vi "Exercise 4.4.vi"() -> ()   [LabVIEW 2020]
uses:
  <vilib>/Analysis/NI_AALBase.lvlib
  <vilib>/Analysis/3filter.llb/Butterworth Filter (DBL).vi
  <vilib>/Analysis/3filter.llb/Filter Passband Type.ctl
panel:
  in  "high cutoff freq: fh":dbl=39.0 format="%0.2f"
  in  "low cutoff freq:":dbl=39.105000000000004 format="%0.4f"
  in  "filter type":T1(ring)=enum."Highpass"
  out "After Filter":dbl[](graph)=[0.0, 0.6054086429729769, 0.8743542473216894, 0.8013797269204491, 0.4638808588516081, 0.0016208481319575085, -0.7580045163981852, -1.221080704726118, -1.329532694477237, -1.1061098691588231, -0.6516319292362134, -0.11925564860102078, 0.32685999298529467, 0.5564986300116397, 0.5088507193494789, 0.20814252119149446, 0.09101816130337614, -0.1485564077005146, -0.33989613656747075, -0.3562115337532852, -0.1465290434450428, 0.25429860374541846, 0.7402352033883393, 1.1689734714393074, 1.4068707655788693, 1.3707775671677735, 0.7183939026271382, -0.02378501952343859, -0.7439605231291739, -1.3067169263115561, -1.5975533640721071, -1.5611303423708822, -1.2218648739986673, -0.6807400423537864, -0.0892023602907166, 0.392241843978935, 0.9747905946845299, 1.1516407043041998, 0.9756730464254995, 0.5729848442452745, 0.11098713644940972, -0.24573581881058892, -0.3791057495877945, -0.24812790449548405, 0.10250586104614756, 0.5582875535009255, 0.6344471555954394, 0.6455591142873733, 0.48400098640909106, 0.12240784296500251, -0.38326601770784574, -0.9148509660653827, -1.330873613656589, -1.5117920518294774, -1.3982830154138846, -1.011383724003272, -0.11245099671986836, 0.699127866764331, 1.290671966311153, 1.5639464946876167, 1.4887900730129608, 1.1166858255338745, 0.5701186035389831, 0.010709133386347602, -0.40462549572607553, -0.5666931257540841, -0.7798171095228799, -0.6449402022246447, -0.30584524569489124, 0.0638598209055572, 0.3065194772758213, 0.32172053026231895, 0.09122719564693194, -0.31960417555827547, -0.7842854006191136, -1.1549575821664675, -0.9716848974061367, -0.6248049854127773, -0.1112553153230218, 0.49351598872918423, 1.0625215391203886, 1.4590885653051924, 1.5811763084677413, 1.3950938998355458, 0.9487112076214625, 0.3602901892843722, -0.5499548756361361, -1.1793384767437638, -1.448404037978766, -1.353116812147694, -0.9709755135184519, -0.4431360698914588, 0.062424387897631384, 0.39606152546676743, 0.46680493564390435, 0.2661164008977511, 0.2042795021341143, -0.037447412047102946, -0.2840706890878546, -0.38899305636335657, -0.2719014040368761, 0.06253488645273242, 0.5304233149454909, 0.9970650539647679, 1.3196700846959315, 1.3918800500063293, 0.8409397850988656, 0.16458234668008975, -0.5440146795184788, -1.152429963955388, -1.532611620363828, -1.603042021021695, -1.3569444419774364, -0.8681744369705768, -0.2730165108341076, 0.2668103317000958, 0.9452861029728707, 1.2274247919967265, 1.1351995962403318, 0.7701083132483948, 0.2884590558210576, -0.13952611752000887, -0.37503739127850366, -0.34731145732281865, -0.07093160056906811, 0.36124613441915354, 0.4713204662877586, 0.5639429496210233, 0.5076731374224686, 0.24438843029636426, -0.19867147752246206, -0.7216223036343026, -1.1855066985653462, -1.4567954079786336, -1.4497607779953885, -1.1543317659623957, -0.30514007223777906, 0.5129623938012557, 1.1653945094064335, 1.536140642788311, 1.5665717572613662, 1.2773319026936516, 0.7667035679648304, 0.18581139586084028, -0.30215134363843443, -0.5667772197468339, -0.8824320879312736, -0.8201094495847365, -0.5023992064809693, -0.09666304430812112, 0.2289186079699732, 0.349710835718934, 0.21663448212310765, -0.13340979582189183, -0.5916899453937949, -1.0122170838048081, -0.9204930537925069, -0.6801144482390487, -0.2569100038548642, 0.3000617513186674, 0.8777755193918795, 1.337014801017256, 1.5574323057436814, 1.4766151402625134, 1.1116853174398322, 0.5571125135893666, -0.3767760073843336, -1.0803885033494895, -1.4525862224711927, -1.4592096346216543, -1.1479894750072646, -0.6393656849896363, -0.09570251481715264, 0.322225960384654, 0.4988279539245859, 0.3946441027584082, 0.3917691025978004, 0.15423861387455107, -0.14417947709129542, -0.3417586970847335, -0.33112098842195525, -0.08584067321812405, 0.33623209306900304, 0.8137811782778508, 1.200830541807984, 1.3721977205576223, 0.9261638564651387, 0.329818982768606, -0.34703088123662806, -0.9812377113052912, -1.43721594492008, -1.6113078735511, -1.4664573765969369, -1.046945867566608, -0.46882753526764986, 0.11115585846157039, 0.8752546495596835, 1.2634724545095883, 1.2667968993057865, 0.958815856074775, 0.47915561105457094, -0.0025427651676084295, -0.33177990059021134, -0.41041528513044545, -0.22196420128901018, 0.16640118626815648, 0.28957712574973193, 0.44838820927464895, 0.4920603860958954, 0.33327813221718816, -0.031243888382397333, -0.5245622076947978, -1.0163750928149309, -1.3649954138424913, -1.4621070540134706, -1.2672179810104716, -0.4855923101464228, 0.3176539963448566, 1.0122792805409193, 1.4699433411458775, 1.606628528311827, 1.4119422158752641, 0.9565479263984091, 0.3754365100977832, -0.16813472210417402, -0.5275151712425132, -0.9493930056056952, -0.9737341367292887, -0.6978140923741032, -0.2767876956877062, 0.11669836680940016, 0.33817439083521883, 0.3091516140181061, 0.03613677930890269, -0.39463826045851524, -0.8452188291913396, -0.8323282018333398, -0.6965358371854609, -0.37312096741695355, 0.11800628400572988, 0.6830537128478369, 1.1865046409287237, 1.4950976135394942, 1.5206637982229037, 1.2492507700335977, 0.7480120715607805, -0.18830385590017684, -0.9493962279489672, -1.4173364959261567, -1.5299988560744744, -1.3041402052124642, -0.8352664993448418, -0.2741310409917075, 0.2133884621355442, 0.4913727748666008, 0.49074889096951213, 0.5633617748052927, 0.35119717436044184, 0.02061363307737052, -0.257266889749427, -0.35161043062743014, -0.20532642562357317, 0.1526516628782142, 0.6197296744892453, 1.0529901555480388, 1.3137524358027015, 0.9741854646532984, 0.47028043478979464, -0.15515819229307343, -0.7939995475917545, -1.3093043298147427, -1.5800856229721347, -1.5410444692106378, -1.205555510915536, -0.6651300594276801, -0.06549983526894998, 0.7698466839591114, 1.2601017462916366, 1.366448027944, 1.1323808568836915, 0.6759363737045065, 0.15997435524365766, -0.25099746129453493, -0.4349639720921017, -0.34467337506899387, -0.018625284736814907, 0.09627934834283103, 0.3032811540993876, 0.4375296346842922, 0.38525204592401985, 0.11205317804639314, -0.3317988747242602, -0.8304514114135069, -1.2402194488196825, -1.4349257019886181, -1.3455708794533692, -0.6465926796292107, 0.12103415373141324, 0.8374723643437596, 1.368010223559577, 1.6073437400168498, 1.5150968444655337, 1.1320106394225853, 0.5719548779635879, -0.007963458302266524, -0.45047682872588357, -0.9779903837309027, -1.0996139786497707, -0.8842070604686469, -0.4692486471159194, -0.025612975095689272, 0.28758161578592034, 0.3650554894208278, 0.182207856082238, -0.20106715329787095, -0.6606895595414763, -0.710741528650062, -0.673407069102057, -0.45520598742029805, -0.04531559681706554, 0.486201079548954, 1.0136216525562451, 1.3966831654800735, 1.5254646223781219, 1.3558645519301393, 0.9252970645788583, 0.007867633037984767, -0.7916396791139617, -1.3440753693237246, -1.5626326312198238, -1.4331365989547127, -1.02294583334103, -0.465672426599566, 0.07393401379620901, 0.4447397262445687, 0.5505586947368704, 0.7121440653004, 0.5454928386085078, 0.20366916100021504, -0.13892177907156888, -0.3325441896484618, -0.2911082784625254, -0.012921516462402138, 0.4227288783506795, 0.8821054181862111, 1.2188989660906735, 0.98306983736249, 0.5803075362410581, 0.02387286509102926, -0.598259272599921, -1.1540303162071952, -1.5106332075766922, -1.5777006119672041, -1.3376130003409799, -0.8540150751230104, -0.256039310540328, 0.6333090812895308, 1.217448471857372, 1.4301380475683017, 1.2838103989146514, 0.870873066446908, 0.3414774450323197, -0.13594479022546047, -0.4199684548816105, -0.43411518273339, -0.18637858192955803, -0.1007849190937869, 0.13446813187695175, 0.346277921259325, 0.3982161477547985, 0.22544629789914916, -0.15109871924303464, -0.6352265000058432, -1.0874947234469232, -1.3693118557106114, -1.3862336311780412, -0.7816544926202527, -0.06897534113248405, 0.6480167131991552, 1.2344481646984766, 1.5686885766077596, 1.582639699316573, 1.2860223327379554, 0.7674487950261693, 0.1719091643452879, -0.3387660589341399, -0.967072036930196, -1.192677289698167, -1.0540683576052041, -0.6662916670223522, -0.19228170868979344, 0.19997088817620856, 0.3820937470466297, 0.29891824611658446, -0.018775583541323027, -0.46606393979866123, -0.5606317485687642, -0.6116599996335546, -0.4998578670104701, -0.1833236696836994]
  out "Before":dynamicdata(graph)=[{"t0"=timestamp(0 s since 1904-01-01), "dt"=0.001, "Y"=array[400 elements], "attributes"=variant("NI_ChannelName"=variant(string "Sine"), "NI_ExpIsRelativeTime"=variant(bool TRUE), "NI_ExpStartTimeStamp"=variant(timestamp timestamp(3810316913.5753865 s since 1904-01-01)), "NI_ExpTimeStamp"=variant(timestamp timestamp(3810316913.5753865 s since 1904-01-01)), "NI_ExpXDimension"=variant(string "t"))}]
  in  "# of Samples":i32=400
  in  "error in (no error) 2":errorcluster caption="error in (no error)"
  in  "Trials":i32=1
  in  "Seed Number":dbl=-1.0
  in  "Noise amplitude":dbl=0.6
  in  "Reset Signal":bool
  in  "error in (no error)":errorcluster
  in  "Duty Cycle (%)":dbl=50.0
  in  "Phase":dbl
  in  "Amplitude":dbl=1.0
  in  "Frequency":dbl=87.1
  in  "Offset":dbl
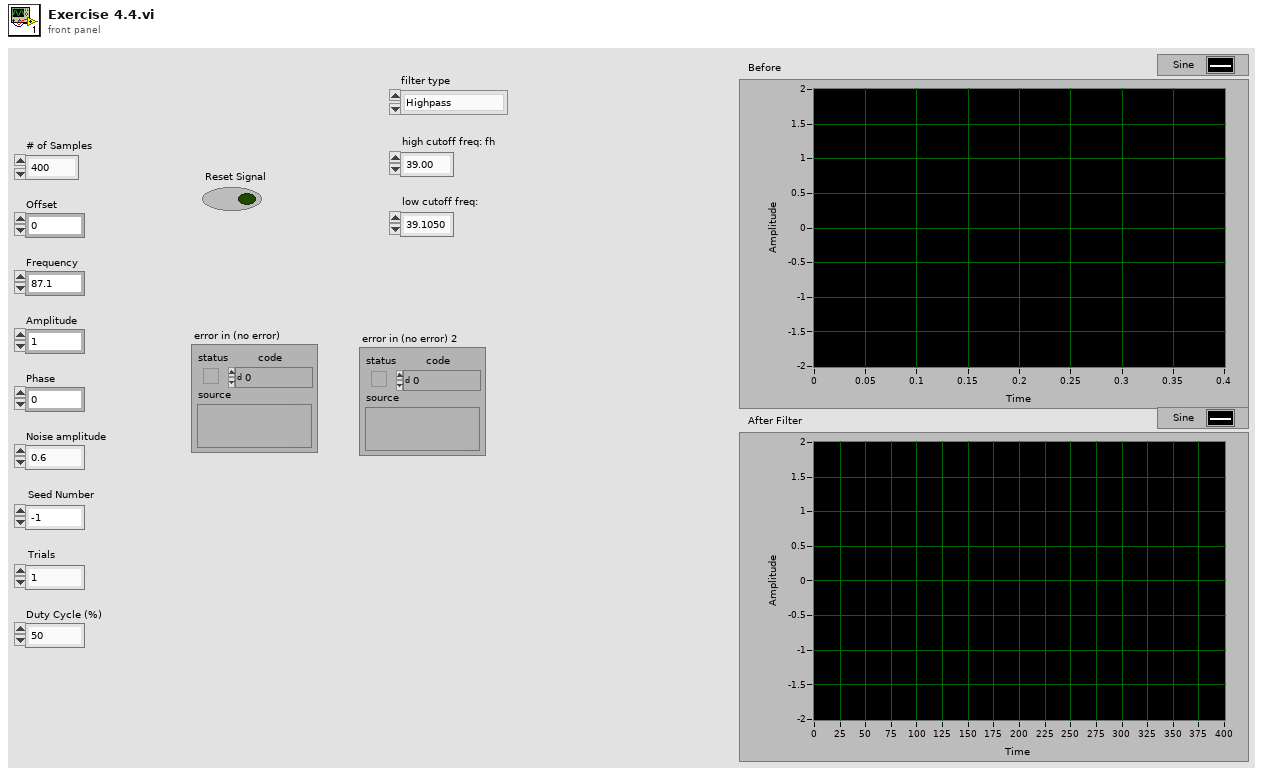
[diagram p1: front panel]
types:
  T1 = enum32{"Lowpass", "Highpass", "Bandpass", "Bandstop"}
  T2 = typedef "NI_AALBase.lvlib/Filter Passband Type.ctl" = enum32{"Lowpass", "Highpass", "Bandpass", "Bandstop"}
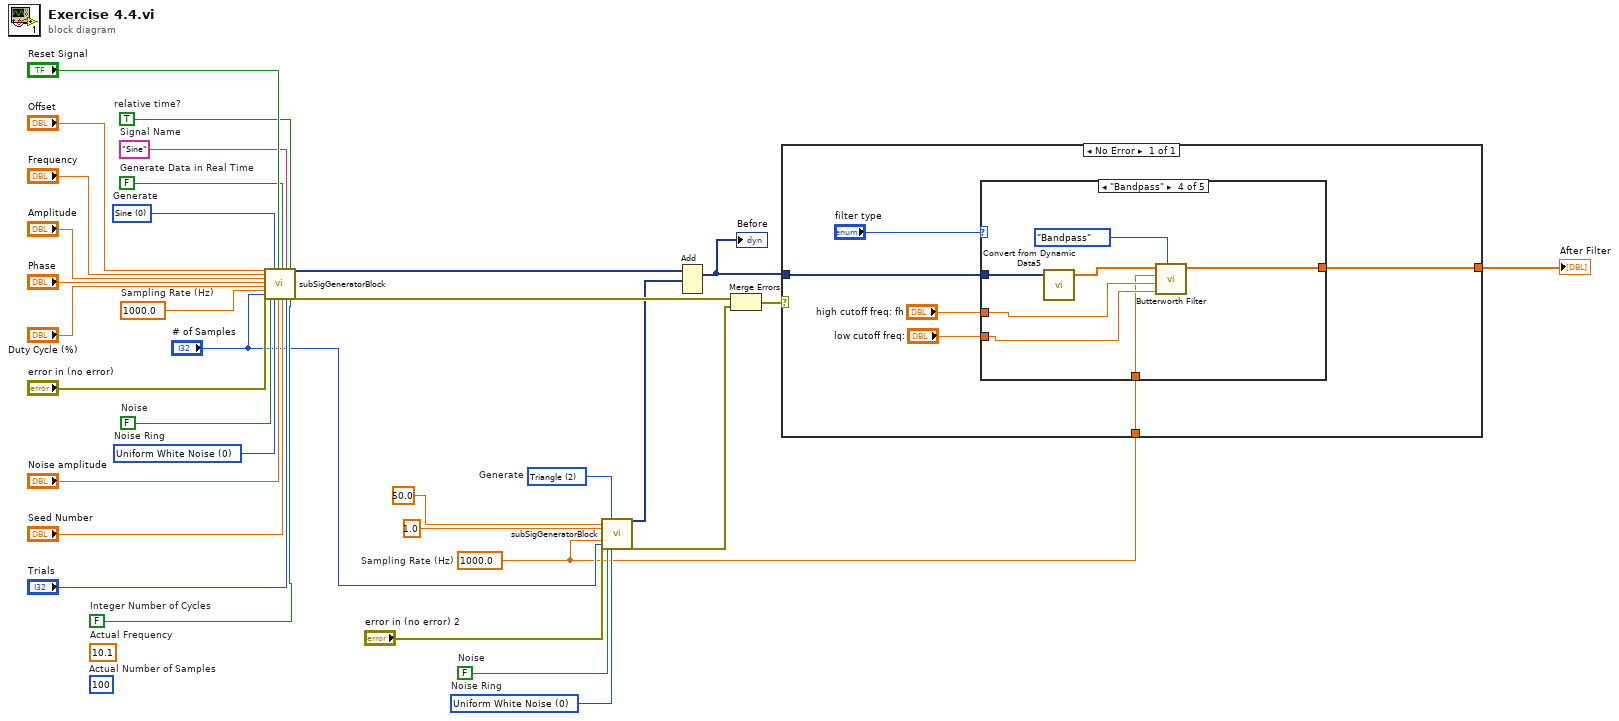
[diagram p0: block diagram]
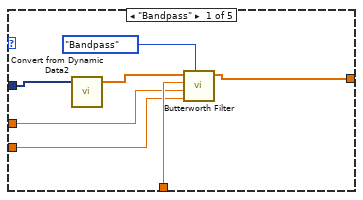
[diagram p2: hidden frame]
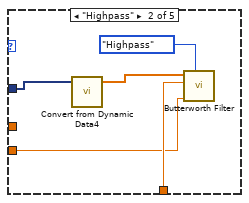
[diagram p3: hidden frame]
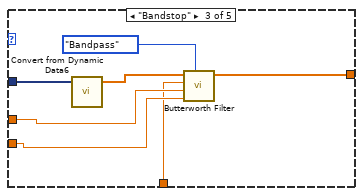
[diagram p4: hidden frame]
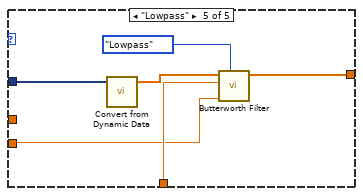
[diagram p5: hidden frame]
diagram:
  w10 = u16 0 items=["Uniform White Noise", "Gaussian White Noise", "Periodic Random Noise", "Gamma Noise", "Poisson Noise", "Binomial Noise", "Bernoulli Noise", "MLS Sequence "]  # Noise Ring
  w11 = FALSE  # Noise
  w12 = u16 2 items=["Sine", "Square", "Triangle", "Sawtooth", "DC"]  # Generate
  w1 = 1000.0  # Sampling Rate (Hz)
  (unwired) 10.1  # Actual Frequency
  (unwired) 100  # Actual Number of Samples
  w16 = FALSE  # Integer Number of Cycles
  w20 = u16 0 items=["Uniform White Noise", "Gaussian White Noise", "Periodic Random Noise", "Gamma Noise", "Poisson Noise", "Binomial Noise", "Bernoulli Noise", "MLS Sequence "]  # Noise Ring
  w21 = FALSE  # Noise
  w22 = TRUE  # relative time?
  w23 = "Sine"  # Signal Name
  w24 = FALSE  # Generate Data in Real Time
  w26 = u16 0 items=["Sine", "Square", "Triangle", "Sawtooth", "DC"]  # Generate
  w29 = 1000.0  # Sampling Rate (Hz)
  n1 = call <vilib>:"subSigGeneratorBlock.vi"("Offset"="Offset", "Frequency"="Frequency", "Amplitude"="Amplitude", "Phase"="Phase", "Duty Cycle (%)"="Duty Cycle (%)", "Sampling Rate (Hz)"=w29, "# of Samples"="# of Samples", "error in (no error)"="error in (no error)", "Noise"=w21, "Generate"=w26, "Noise Ring"=w20, "Reset Signal"="Reset Signal", "Noise Amplitude"="Noise amplitude", "Generate Data in Real Time"=w24, "Seed Number"="Seed Number", "Signal Name"=w23, "trials"="Trials", "relative time?"=w22, "Integer Number of Cycles"=w16) -> ("Signal"=w5:dynamicdata, "error out"=w8:errorcluster)  [unwired: 7 in]
  n2 = call <vilib>:"subSigGeneratorBlock.vi"("Frequency"=50.0 ("Frequency 2"), "Amplitude"=1.0 ("Amplitude 2"), "Sampling Rate (Hz)"=w1, "# of Samples"="# of Samples", "error in (no error)"="error in (no error) 2", "Noise"=w11, "Generate"=w12, "Noise Ring"=w10) -> ("Signal"=w6:dynamicdata, "error out"=w9:errorcluster)  [unwired: 18 in]
  n3 = Add(1:w6, 2:w5) -> (0:w3:dynamicdata)  [unwired: 1 in, 1 out]
  "Before" <- w3
  n4 = Merge Errors(w8, w9) -> (w7:errorcluster)
  n5 = case shown="No Error" w7 {
    tunnel: w3 -> [w39]
    tunnel: [w38] -> w2
    tunnel: w1 -> [w37]
    frame No Error {
      n6 = case shown="\"Bandpass\"" "filter type" {
        tunnel: w39 -> [w44 w49 w54 w61 w71]
        tunnel: [w43 _ w52 w59 w68] -> w38
        tunnel: w37 -> [w42 w50 w53 w60 w67]
        tunnel: "high cutoff freq: fh" -> [w41 _ w55 w62 _]
        tunnel: "low cutoff freq:" -> [w40 w47 w56 w63 w66]
        frame "Bandpass" {
          n7 = call "Convert from Dynamic Data2"("Dynamic Data Type"=w44) -> ("Array"=w46:dbl[])  [unwired: 3 in]
          n8 = call-poly <vilib>:"Butterworth Filter.vi"("filter type"=Filter_Passband_Type."Bandpass", "low cutoff freq: fl"=w40, "high cutoff freq: fh"=w41, "sampling freq: fs"=w42, "X"=w46) -> ("Filtered X"=w43:dbl[])  [unwired: 3 in, 1 out]
        }
        frame "Highpass" {
          n9 = call "Convert from Dynamic Data4"("Dynamic Data Type"=w49) -> ("Array"=w51:dbl[])  [unwired: 3 in]
          n10 = call-poly <vilib>:"Butterworth Filter.vi"("filter type"=Filter_Passband_Type."Highpass", "low cutoff freq: fl"=w47, "sampling freq: fs"=w50, "X"=w51) -> ()  [unwired: 4 in, 2 out]
        }
        frame "Bandstop" {
          n11 = call "Convert from Dynamic Data6"("Dynamic Data Type"=w54) -> ("Array"=w58:dbl[])  [unwired: 3 in]
          n12 = call-poly <vilib>:"Butterworth Filter.vi"("filter type"=Filter_Passband_Type."Bandpass", "low cutoff freq: fl"=w56, "high cutoff freq: fh"=w55, "sampling freq: fs"=w53, "X"=w58) -> ("Filtered X"=w52:dbl[])  [unwired: 3 in, 1 out]
        }
        frame "Bandpass" {
          n13 = call "Convert from Dynamic Data5"("Dynamic Data Type"=w61) -> ("Array"=w65:dbl[])  [unwired: 3 in]
          n14 = call-poly <vilib>:"Butterworth Filter.vi"("filter type"=Filter_Passband_Type."Bandpass", "low cutoff freq: fl"=w63, "high cutoff freq: fh"=w62, "sampling freq: fs"=w60, "X"=w65) -> ("Filtered X"=w59:dbl[])  [unwired: 3 in, 1 out]
        }
        frame "Lowpass" {
          n15 = call "Convert from Dynamic Data"("Dynamic Data Type"=w71) -> ("Array"=w70:dbl[])  [unwired: 3 in]
          n16 = call-poly <vilib>:"Butterworth Filter.vi"("filter type"=Filter_Passband_Type."Lowpass", "low cutoff freq: fl"=w66, "sampling freq: fs"=w67, "X"=w70) -> ("Filtered X"=w68:dbl[])  [unwired: 4 in, 1 out]
        }
      }
    }
  }
  "After Filter" <- w2
